vi "TLPM Get Next Fast Array Measurement.vi"(8 "error in (no error)":errorcluster {"code" format="%.0x"}, 11 "instrument handle":refnum<visa-resource-name>) -> (0 "error out":errorcluster {"code" format="%.0x"}, 1 "Timestamps":u32[](array[numeric]), 2 "Count":u16, 3 "instrument handle out":refnum<visa-resource-name>, 4 "Meas Data":dbl[](array[numeric]) format="%.2p")   [LabVIEW 2019]
doc: "This VI is used to obtain measurements from the instrument. \nThe result are timestamp - value pairs.\n\n\nRemark:\nThis VI starts a new measurement cycle and after finishing measurement the result is received. Subject to the actual Average Count this may take up to seconds."
uses:
  TLPM_32.dll
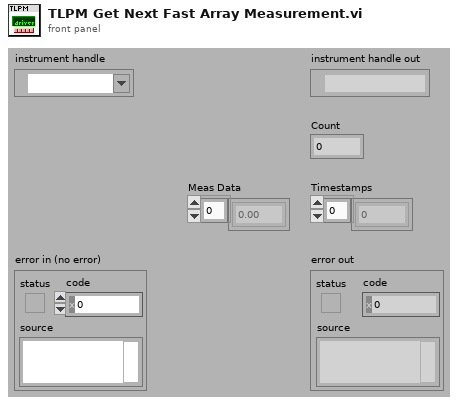
[diagram p1: front panel]
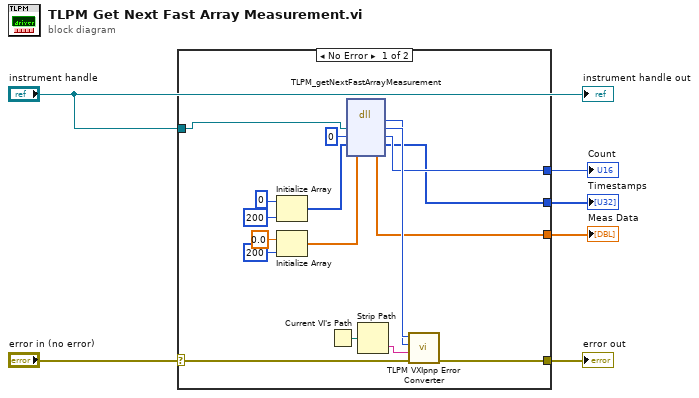
[diagram p0: block diagram]
diagram:
  n1 = case shown="No Error" "error in (no error)" {
    selector: "error in (no error)" -> [w18 w24]
    tunnel: [w17 w24] -> w6
    tunnel: "instrument handle" -> [w22 _]
    tunnel: [w15 _] -> w3
    tunnel: [w11 _] -> w2
    tunnel: [w7 _] -> w1
    frame No Error {
      n2 = Initialize Array(u32 0 ("element"), 200 ("dimension size")) -> (w14:u32[])
      n3 = Initialize Array(0.0 ("element"), 200 ("dimension size")) -> (w10:dbl[])
      n4 = Current VI's Path() -> (path=w23:path)
      n5 = dll-call lib="TLPM_32.dll" fn="TLPM_getNextFastArrayMeasurement"("Instrument Handle"=w22, "Count"=u16 0, "Timestamps"=w14, "Meas Data"=w10) -> (w20:i32, "Instrument Handle"=w21:u32, "Count"=w15:u16, "Timestamps"=w11:u32[], "Meas Data"=w7:dbl[])  [unwired: 3 in, 2 out]
      n6 = Strip Path(path=w23) -> (name=w19:string)  [unwired: 1 out]
      n7 = call "TLPM VXIpnp Error Converter.vi"("error in (no error)"=w18, "Name Of VI (\"\")"=w19, "CVI Error Code (0)"=w20, "instrument handle"=w21) -> ("error out"=w17:errorcluster)  [unwired: 6 in, 1 out]
    }
    frame Error {
    }
  }
  "error out" <- w6
  "Count" <- w3
  "Timestamps" <- w2
  "Meas Data" <- w1
  "instrument handle out" <- "instrument handle"
